vi "CreateMaze.vi"(8 "error in (no error)":errorcluster) -> (0 "error out":errorcluster, 2 "Maze*":refnum<data-value>)   [LabVIEW 2016]
uses:
  Base/Maze/Maze.lvclass
  Base/Room/Direction.ctl
  Base/Door/Door.lvclass
  C:/github/LVOOP-creational-patterns/Maze-Classes/src/Base/MapSite/MapSite.lvclass
  Base/Wall/Wall.lvclass
  Base/Room/Room.lvclass
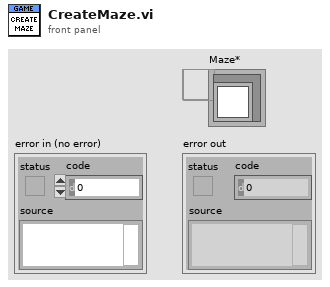
[diagram p1: front panel]
types:
  T1 = typedef "Room.lvclass/Direction.ctl" = enum16{"North", "South", "East", "West"}
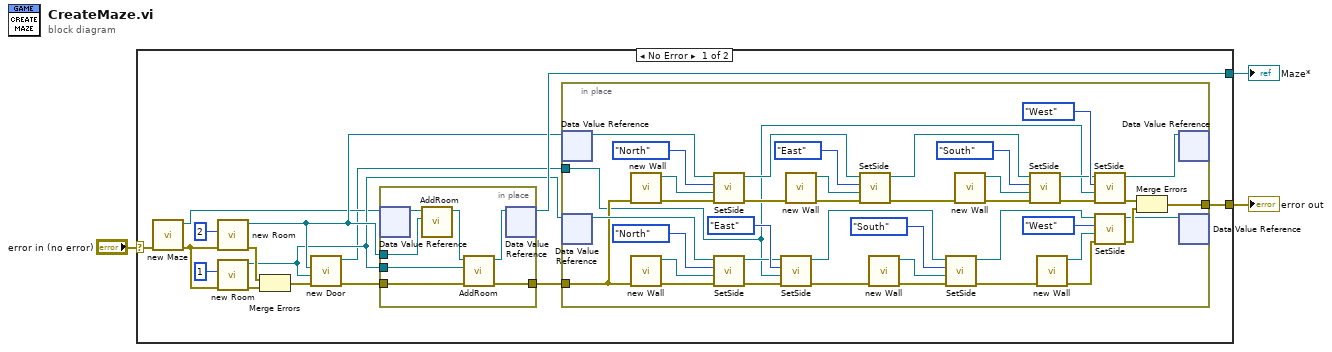
[diagram p0: block diagram]
diagram:
  n1 = case shown="No Error" "error in (no error)" {
    selector: "error in (no error)" -> [w14 w67]
    tunnel: [w12 w67] -> w2
    tunnel: [w13 _] -> w1
    frame No Error {
      n2 = call "new Maze.vi"("error in (no error)"=w14) -> ("error out"=w6:errorcluster, "Maze* out"=w7:refnum<data-value>)  [unwired: 9 in]
      n3 = call "new Room.vi"("error in (no error)"=w6, "roomNumber"=2) -> ("error out"=w10:errorcluster, "Room* out"=w11:refnum<data-value>)  [unwired: 8 in]
      n4 = call "new Room.vi"("error in (no error)"=w6, "roomNumber"=1) -> ("error out"=w8:errorcluster, "Room* out"=w9:refnum<data-value>)  [unwired: 8 in]
      n5 = Merge Errors(w10, w8) -> (w16:errorcluster)
      n6 = call "new Door.vi"("error in (no error)"=w16, "r2"=w9, "r1"=w11) -> ("error out"=w4:errorcluster, "Door* out"=w5:refnum<data-value>)  [unwired: 7 in]
      n7 = in-place {
        in-place-border: w11 -> [w63]
        in-place-border: w9 -> [w62]
        in-place-border: [w61] -> w15
        in-place-border: w4 -> [w60]
        n8 = in-place-dvr #1(w7) -> (w66:refnum<class "Maze.lvclass">)  [unwired: 1 out]
        n9 = call-dynamic "AddRoom.vi"("Room*"=w63, "Maze in"=w66) -> ("Maze out"=w65:refnum<class "Maze.lvclass">)  [unwired: 8 in, 1 out]
        n10 = call-dynamic "AddRoom.vi"("error in (no error)"=w60, "Room*"=w62, "Maze in"=w65) -> ("error out"=w61:errorcluster, "Maze out"=w64:refnum<class "Maze.lvclass">)  [unwired: 7 in]
        n11 = in-place-dvr #1(w64) -> (w13:refnum<data-value>)  [unwired: 1 out]
      }
      n12 = in-place {
        in-place-border: w15 -> [w39]
        in-place-border: [w34] -> w12
        in-place-border: w5 -> [w31]
        n13 = in-place-dvr #2(w11) -> (w41:refnum<class "Room.lvclass">)  [unwired: 1 out]
        n14 = in-place-dvr #3(w9) -> (w40:refnum<class "Room.lvclass">)  [unwired: 1 out]
        n15 = call "new Wall.vi"("error in (no error)"=w39) -> ("error out"=w29:errorcluster, "Wall* out"=w30:refnum<data-value>)  [unwired: 9 in]
        n16 = call "new Wall.vi"("error in (no error)"=w39) -> ("error out"=w27:errorcluster, "Wall* out"=w28:refnum<data-value>)  [unwired: 9 in]
        n17 = call-dynamic "SetSide.vi"("error in (no error)"=w29, "MapSite*"=w30, "Direction"=Direction."North", "Room in"=w41) -> ("error out"=w59:errorcluster, "Room out"=w52:refnum<class "Room.lvclass">)  [unwired: 6 in]
        n18 = call-dynamic "SetSide.vi"("error in (no error)"=w27, "MapSite*"=w28, "Direction"=Direction."North", "Room in"=w40) -> ("error out"=w32:errorcluster, "Room out"=w43:refnum<class "Room.lvclass">)  [unwired: 6 in]
        n19 = call-dynamic "SetSide.vi"("error in (no error)"=w32, "MapSite*"=w31, "Direction"=Direction."East", "Room in"=w43) -> ("error out"=w49:errorcluster, "Room out"=w44:refnum<class "Room.lvclass">)  [unwired: 6 in]
        n20 = call "new Wall.vi"("error in (no error)"=w59) -> ("error out"=w25:errorcluster, "Wall* out"=w26:refnum<data-value>)  [unwired: 9 in]
        n21 = call-dynamic "SetSide.vi"("error in (no error)"=w25, "MapSite*"=w26, "Direction"=Direction."East", "Room in"=w52) -> ("error out"=w58:errorcluster, "Room out"=w53:refnum<class "Room.lvclass">)  [unwired: 6 in]
        n22 = call "new Wall.vi"("error in (no error)"=w49) -> ("error out"=w21:errorcluster, "Wall* out"=w22:refnum<data-value>)  [unwired: 9 in]
        n23 = call-dynamic "SetSide.vi"("error in (no error)"=w21, "MapSite*"=w22, "Direction"=Direction."South", "Room in"=w44) -> ("error out"=w50:errorcluster, "Room out"=w45:refnum<class "Room.lvclass">)  [unwired: 6 in]
        n24 = call "new Wall.vi"("error in (no error)"=w58) -> ("error out"=w23:errorcluster, "Wall* out"=w24:refnum<data-value>)  [unwired: 9 in]
        n25 = call-dynamic "SetSide.vi"("error in (no error)"=w23, "MapSite*"=w24, "Direction"=Direction."South", "Room in"=w53) -> ("error out"=w33:errorcluster, "Room out"=w54:refnum<class "Room.lvclass">)  [unwired: 6 in]
        n26 = call "new Wall.vi"("error in (no error)"=w50) -> ("error out"=w19:errorcluster, "Wall* out"=w20:refnum<data-value>)  [unwired: 9 in]
        n27 = call-dynamic "SetSide.vi"("error in (no error)"=w33, "MapSite*"=w31, "Direction"=Direction."West", "Room in"=w54) -> ("error out"=w38:errorcluster, "Room out"=w36:refnum<class "Room.lvclass">)  [unwired: 6 in]
        n28 = call-dynamic "SetSide.vi"("error in (no error)"=w19, "MapSite*"=w20, "Direction"=Direction."West", "Room in"=w45) -> ("error out"=w37:errorcluster, "Room out"=w35:refnum<class "Room.lvclass">)  [unwired: 6 in]
        n29 = Merge Errors(w38, w37) -> (w34:errorcluster)
        n30 = in-place-dvr #2(w36) -> ()  [unwired: 2 out]
        n31 = in-place-dvr #3(w35) -> ()  [unwired: 2 out]
      }
    }
    frame Error {
    }
  }
  "error out" <- w2
  "Maze*" <- w1
